vi "OC2 gui.vi"() -> ()   [LabVIEW 2009]
uses:
  Instance           2 15Saved   TCM gui .vi
  Instance           1 15Saved   TCM gui .vi
panel:
  in  "read setpoint":bool
  in  "Rate deg/s":dbl format="%.3f"
  out "error out":errorcluster
  in  "temp data":dbl[][](graph)
  in  "error in":errorcluster
  in  "VISA resource name":refnum<visa-resource-name>
  out "Control":enum16{"Off", "On"}(ring)
  in  "program\n  stop":bool
  in  "Continuous":bool
  in  "Update":bool
  out "Temperature":dbl format="%.3f"
  out "Setpoint":dbl format="%.3f"
  in  "write output control drive":bool
  in  "Control  Output":u16(ring) items=["Off", "On"]
  in  "write sensor":bool
  in  "value":dbl format="%.3f"
  in  "Setpoint control":u16(ring) items=["Pot", "Value"]
  # "GUI Control"
  # "Report"
  # "V1.02"
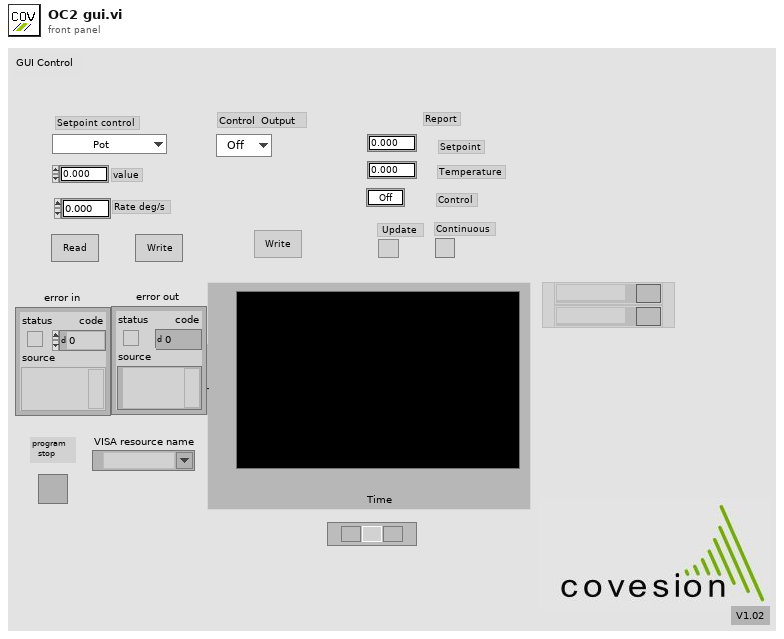
[diagram p1: front panel]
types:
  T1 = cluster{"Setpoint control":u16, "value":dbl, dbl, dbl, dbl, "Rate deg/s":dbl, dbl}
  T2 = cluster{"Setpoint":u16, "pot range":dbl, "value":dbl, "pot offset":dbl, "X coeff deg/V":dbl, "Rate deg/V":dbl, "C coeff deg":dbl}
  T3 = cluster{"Setpoint":dbl, "Temperature":dbl, "Control":i32, "Output %":dbl, "Alarms":i32, "Faults":i32, "TEMP OK":i32, "Supply VDC":dbl, "Version":dbl, "Test cycle":i32, "Test Mode":i32, "Checksum":i32}
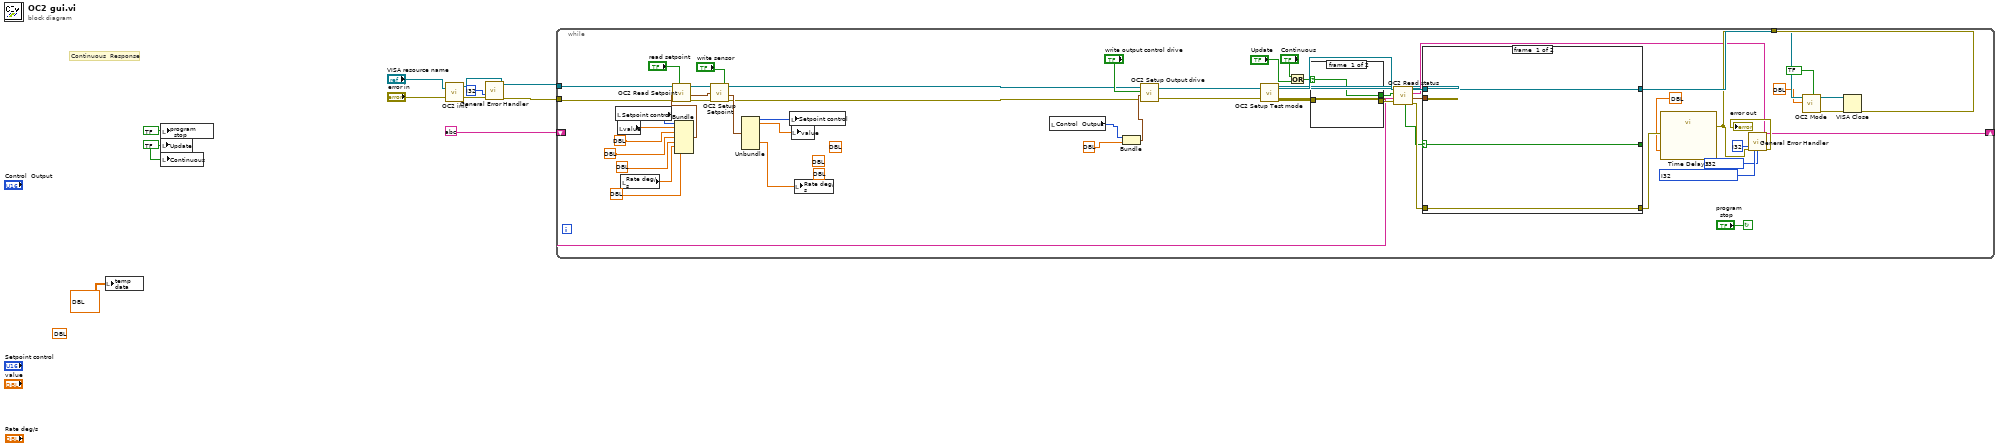
[diagram p0: block diagram]
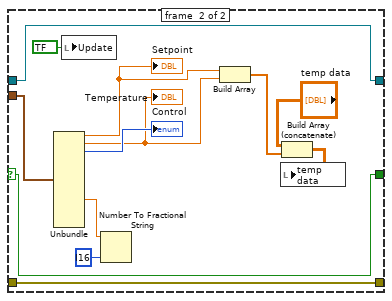
[diagram p2: hidden frame]
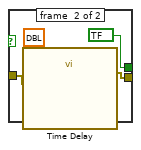
[diagram p3: hidden frame]
diagram:
  w16 = bool ? ("Update")
  (unwired) dbl ? ("data loop")
  # "Continuous  Response"
  n1 = local write "temp data"(dbl[][] ? ("appended array")) -> ()
  n2 = local write "Update"(w16) -> ()
  n3 = local write "program\n  stop"(bool ? ("program\n  stop")) -> ()
  n4 = local write "Continuous"(w16) -> ()
  n5 = call "OC2 init.vi"("error in (no error)"="error in", "VISA resource name"="VISA resource name") -> ("error out"=w9:errorcluster, "duplicate VISA resource name"=w11:refnum<visa-resource-name>)
  n6 = call <vilib>:"General Error Handler.vi"("type of dialog (OK msg:1)"=i32 ?, "error in (no error)"=w9) -> ("error out"=w10:errorcluster)  [unwired: 9 in, 4 out]
  n7 = while {
    tunnel: w10 -> [w26]
    tunnel: w11 -> [w27]
    tunnel: [w55] -> w6
    tunnel: [w46] -> w7
    shift-right: [w40] -> _
    shift-left: string ? -> [w41]
    stop <- "program\n  stop" continue-if-true
    (unwired) dbl ?
    (unwired) dbl ?
    (unwired) dbl ?
    w47 = i32 ? items=["no exception", "cancel error on match", "set error on match"] ("[exception action] (none:0)")
    n8 = local read "Setpoint control"() -> (w63:u16)
    n9 = local read "value"() -> (w64:dbl)
    n10 = local read "Rate deg/s"() -> (w30:dbl)
    n11 = Bundle("Setpoint control"=w63, "value"=w64, dbl ?, dbl ?, dbl ?, "Rate deg/s"=w30, dbl ?) -> (w33:T1)  [unwired: 1 in]
    n12 = call "OC2 Read Setpoint.vi"("enable"="read setpoint", "error in (no error)"=w26, "Read  setpoint values"=w33, "VISA resource name"=w27) -> ("error out"=w34:errorcluster, "Read  setpoint values out"=w35:T2, "dup VISA resource name"=w32:refnum<visa-resource-name>)  [unwired: 5 in]
    n13 = call "OC2 Setup Setpoint.vi"("VISA resource name"=w32, "Setup setpoint values in"=w35, "error in (no error)"=w34, "enable"="write sensor") -> ("dup VISA resource name"=w22:refnum<visa-resource-name>, "Setup setpoint values out"=w36:T2, "error out"=w21:errorcluster)
    n14 = Unbundle(w36) -> ("Setpoint"=w38:u16, "pot range"=w37:dbl, "Rate deg/V"=w31:dbl)  [unwired: 4 out]
    n15 = local write "Setpoint control"(w38) -> ()
    n16 = local write "value"(w37) -> ()
    n17 = local write "Rate deg/s"(w31) -> ()
    n18 = local read "Control  Output"() -> (w25:u16)
    n19 = Bundle("Control  Output"=w25, dbl ?) -> (w23:cluster{"Control  Output":u16, dbl})  [unwired: 1 in]
    n20 = call "OC2 Setup Output drive.vi"("error in (no error)"=w21, "control output values"=w23, "write control output"="write output control drive", "VISA resource name"=w22) -> ("error out"=w28:errorcluster, "dup VISA resource name"=w29:refnum<visa-resource-name>)
    n21 = call "OC2 Setup Test mode.vi"("error in (no error)"=w28, "VISA resource name"=w29) -> ("error out"=w60:errorcluster, "dup VISA resource name"=w56:refnum<visa-resource-name>)  [unwired: 2 in]
    n22 = Or(x="Continuous", y="Update") -> (x .or. y?=w52:bool)
    n23 = case shown="True" w52 {
      selector: w52 -> [w83 _]
      tunnel: [w83 bool ?] -> w49
      tunnel: w60 -> [w82 w86]
      tunnel: [w82 w87] -> w57
      frame #0 {
      }
      frame #1 {
        n24 = call "Time Delay"("error in (no error)"=w86, "Delay Time (s)"=dbl ?) -> ("error out"=w87:errorcluster)  [unwired: 9 in]
      }
    }
    n25 = call "OC2 Read status.vi"("VISA resource name"=w56, "enable"=w49, "feedback read buffer"=w41, "error in"=w57) -> ("RX packet ok"=w42:bool, "dup VISA resource name"=w58:refnum<visa-resource-name>, "feedback buffer"=w40:string, "Report cluster"=w44:T3, "error out"=w59:errorcluster)
    n26 = case shown="True" w42 {
      selector: w42 -> [w66 w75]
      tunnel: [w67 w77] -> w55
      tunnel: [w68 w78] -> w54
      tunnel: w59 -> [w68 w78]
      tunnel: w58 -> [w67 w77]
      tunnel: [w66 w75] -> _
      tunnel: w44 -> [_ w72]
      frame #0 {
      }
      frame #1 {
        n27 = Unbundle(w72) -> ("Setpoint"=w80:dbl, "Temperature"=w71:dbl, "Control"=→"Control":i32, "Version"=w70:dbl)  [unwired: 8 out]
        "Setpoint" <- w80
        "Temperature" <- w71
        n28 = local write "Update"(bool ? ("Update")) -> ()
        n29 = Number To Fractional String(number=w70, precision (6)=i16 ?) -> ()  [unwired: 2 in, 1 out]
        n30 = Build Array(w80, w71) -> (w76:dbl[])
        n31 = Build Array (concatenate)("temp data", w76) -> (w74:dbl[][])
        n32 = local write "temp data"(w74) -> ()
      }
    }
    n33 = call "Time Delay3"("error in (no error)"=w54, "Delay Time (s)"=dbl ?) -> ("error out"=w46:errorcluster)  [unwired: 9 in]
    n34 = call <vilib>:"General Error Handler.vi"("type of dialog (OK msg:1)"=i32 ?, "error in (no error)"=w46, "[exception action] (none:0)"=w47, "[exception code]"=i32 ?) -> ("error out"=→"error out":errorcluster)  [unwired: 7 in, 4 out]
  }
  n35 = call "OC2 Mode.vi"("coms"=bool ?, "error in (no error)"=w7, "mode channel 1"=dbl ? ("mode channel 2"), "VISA resource in"=w6) -> ("error out"=w5:errorcluster, "VISA resource out"=w4:refnum<visa-resource-name>)  [unwired: 6 in]
  n36 = VISA Close(VISA resource name=w4, error in (no error)=w5) -> ()  [unwired: 1 out]
